vi "Check Uneven Quadrature Input.vi"(10 "X In":dbl[](array[numeric]), 11 "T":dbl[](array[numeric])) -> (0 "error":i32, 2 "X Out":dbl[](array[numeric]), 3 "delta T":dbl[](array[numeric]))   [LabVIEW 2014, in "NI_AALPro.lvlib"]
uses:
  NI_AALPro.lvlib
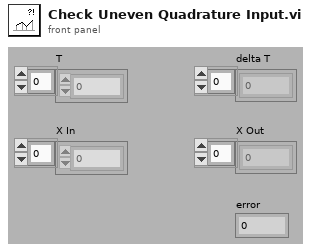
[diagram p1: front panel]
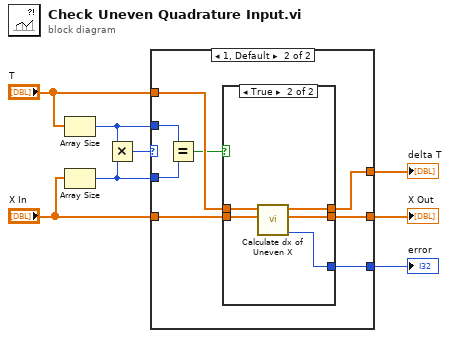
[diagram p0: block diagram]
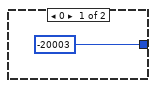
[diagram p2: hidden frame]
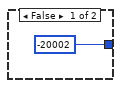
[diagram p3: hidden frame]
diagram:
  n1 = Array Size(array="T") -> (size(s)=w4:i32)
  n2 = Array Size(array="X In") -> (size(s)=w3:i32)
  n3 = Multiply(x=w4, y=w3) -> (x*y=w2:i32)
  n4 = case shown="1, Default" w2 {
    tunnel: w4 -> [_ w13]
    tunnel: "X In" -> [_ w16]
    tunnel: [_ w14] -> w1
    tunnel: [_ w15] -> w5
    tunnel: w3 -> [_ w10]
    tunnel: "T" -> [_ w17]
    tunnel: [-20003 ("error") w11] -> w8
    frame 0 {
    }
    frame 1, Default {
      n5 = Equal?(x=w13, y=w10) -> (x = y?=w12:bool)
      n6 = case shown="True" w12 {
        tunnel: w17 -> [_ w20]
        tunnel: w16 -> [_ w23]
        tunnel: [_ w22] -> w15
        tunnel: [_ w21] -> w14
        tunnel: [-20002 ("f") w19] -> w11
        frame False {
        }
        frame True {
          n7 = call "Calculate dx of Uneven X.vi"("Y In"=w23, "X"=w20) -> ("error"=w19:i32, "Y out"=w21:dbl[], "delta X"=w22:dbl[])  [unwired: 7 in]
        }
      }
    }
  }
  "delta T" <- w5
  "X Out" <- w1
  "error" <- w8
